vi "DAQ_basics.vi"() -> ()   [LabVIEW 2016]
uses:
  <vilib>/DAQmx/write.llb/DAQmx Write.vi
  <vilib>/DAQmx/write.llb/DAQmx Write (Digital 1D Wfm NChan NSamp).vi
  <vilib>/DAQmx/create/channels.llb/DAQmx Create Channel (DO-Digital Output).vi
  <vilib>/DAQmx/configure/timing.llb/DAQmx Timing (Sample Clock).vi
  <vilib>/DAQmx/create/channels.llb/DAQmx Create Channel (AI-Voltage-Basic).vi
  <vilib>/DAQmx/read.llb/DAQmx Read (Analog Wfm 1Chan NSamp).vi
  <vilib>/Waveform/DWDTOps.llb/DWDT Get Waveform Time Array.vi
panel:
  in  "Pre-sampling (ms)":dbl=300.0 format="%#_13g"
  in  "Stim parameters":T1={"Name"="", "VPs"=[], "Concentrations (ppm)"=[], "Back valve ON delays"=[], "Back valve OFF delays"=[], "Pulse duration (ms)"=250.0, "Step duration (ms)"=2.0, "Sampling rate (Hz)"=20000.0}
  out "data":waveform(dbl)(graph)
  out "error out":errorcluster
  in  "Back valves":tag[](array[tag])
  in  "Odour valves":tag[](array[tag])
  in  "Counter valves":tag[](array[tag])
  in  "error in":errorcluster
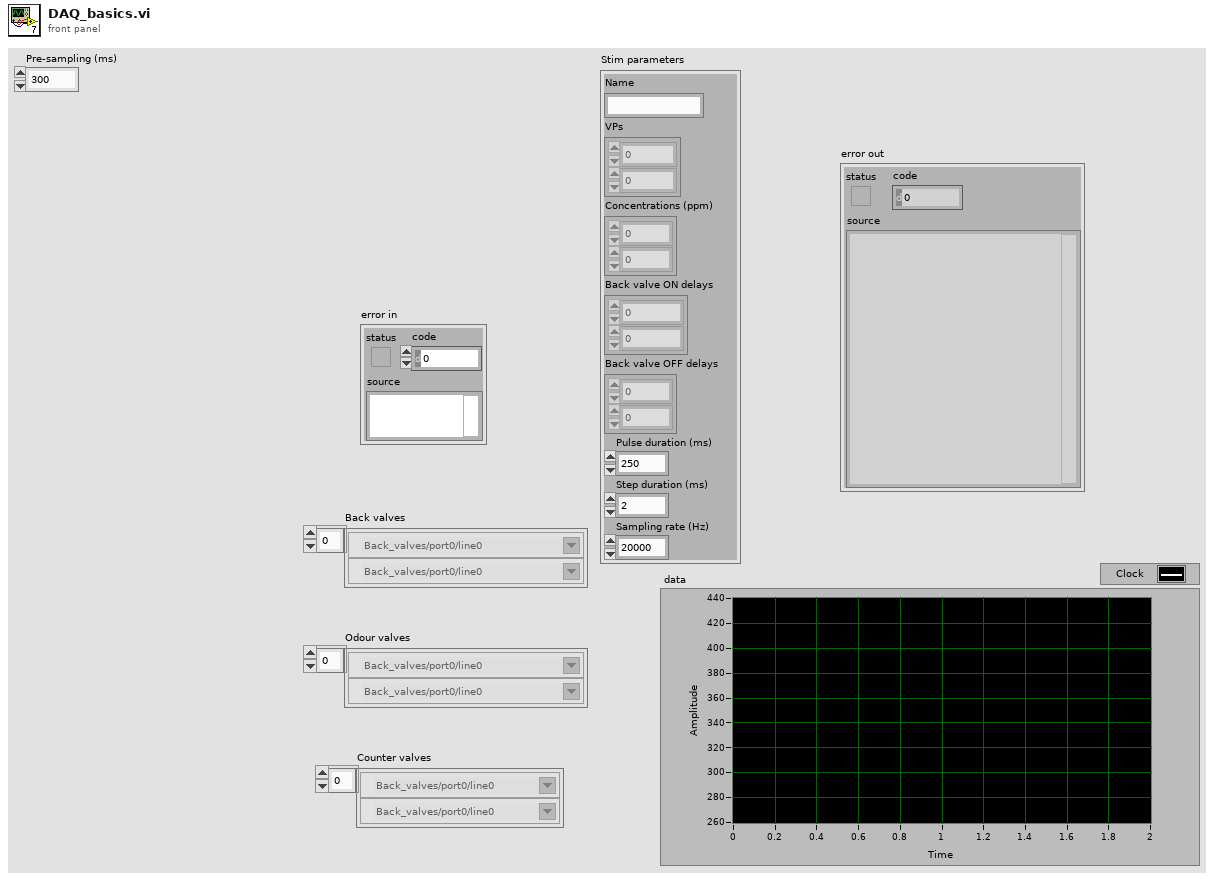
[diagram p1: front panel]
types:
  T1 = cluster{"Name":string, "VPs":dbl[], "Concentrations (ppm)":dbl[], "Back valve ON delays":dbl[], "Back valve OFF delays":dbl[], "Pulse duration (ms)":dbl, "Step duration (ms)":dbl, "Sampling rate (Hz)":dbl}
  T2 = cluster{"VISA Refnum in":refnum<visa-resource-name>, "error in (no error)":errorcluster}
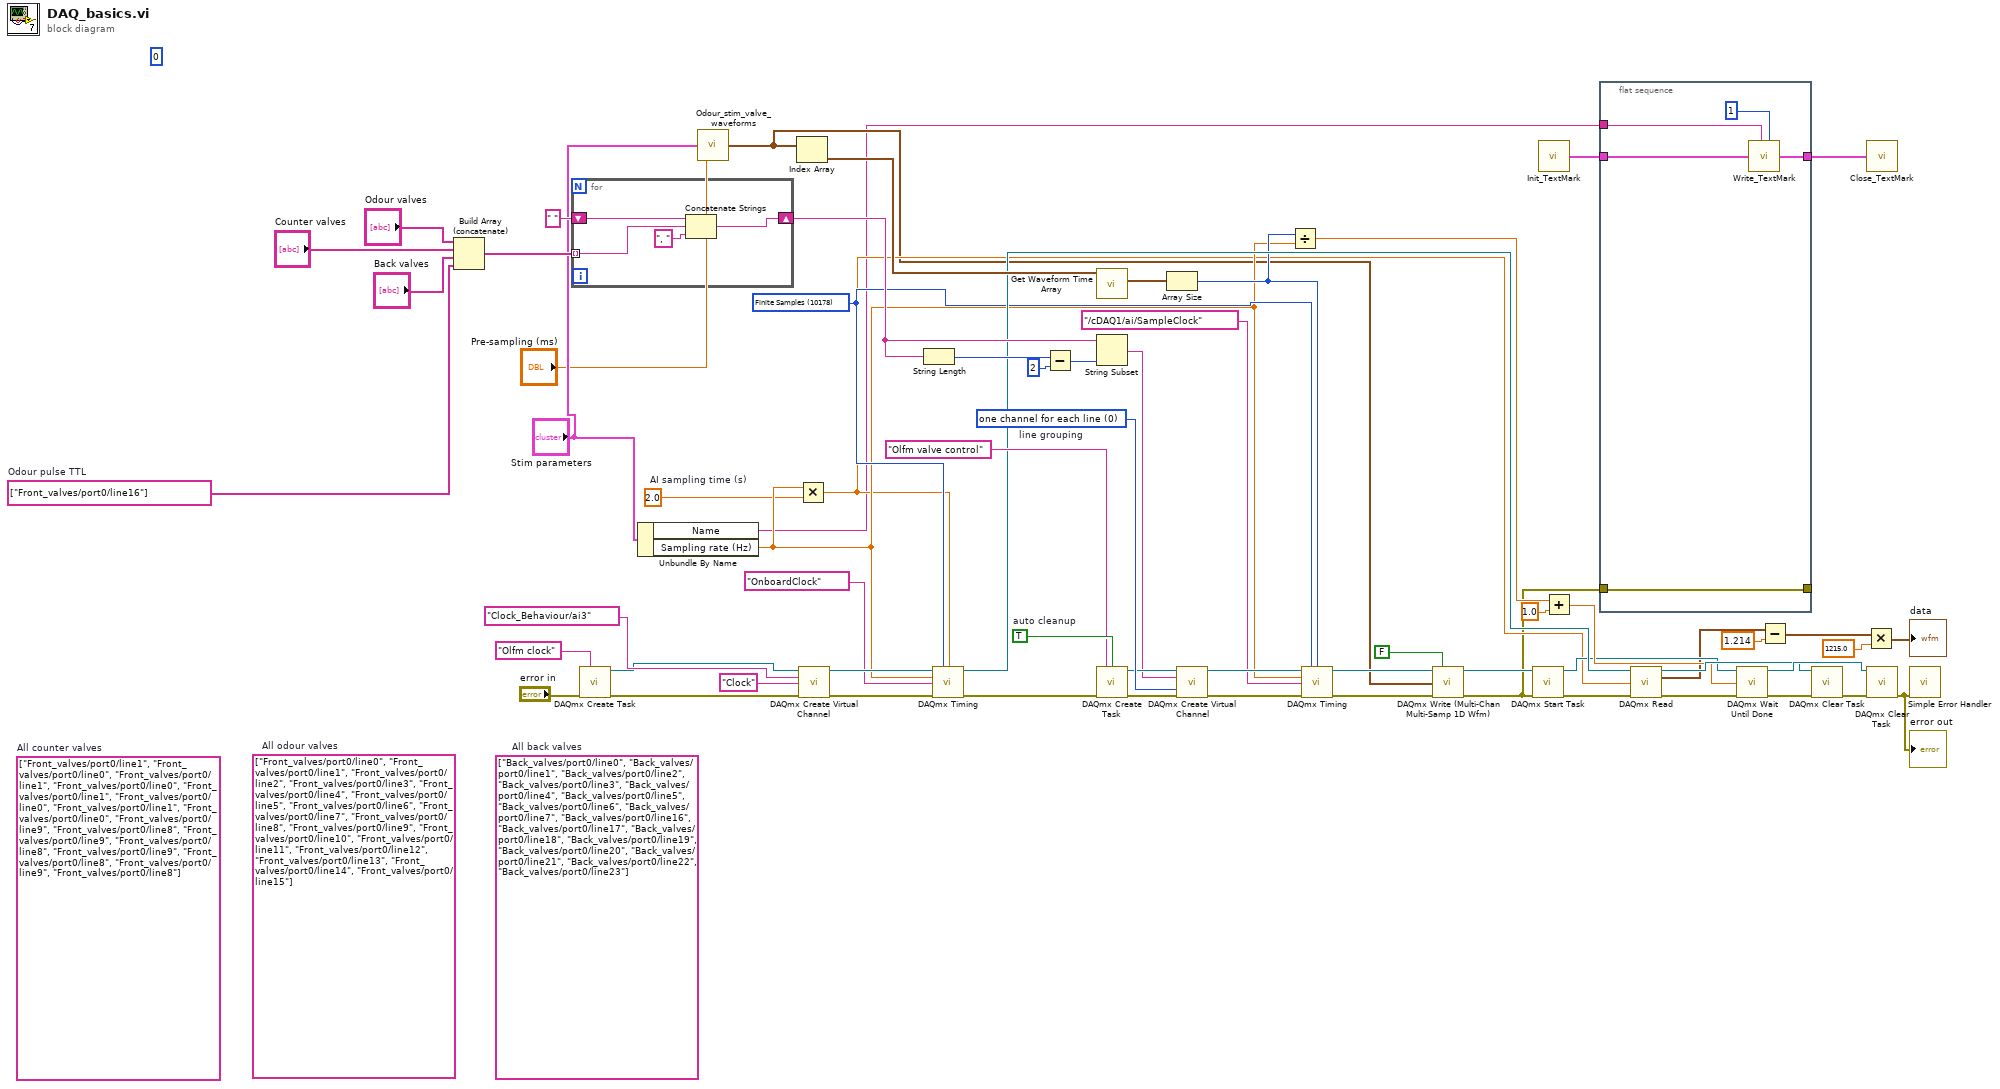
[diagram p0: block diagram]
diagram:
  (unwired) tag[] ["Back_valves/port0/line0", "Back_valves/port0/line1", "Back_valves/port0/line2", "Back_valves/port0/line3", "Back_valves/port0/line4", "Back_valves/port0/line5", "Back_valves/port0/line6", "Back_valves/port0/line7", "Back_valves/port0/line16", "Back_valves/port0/line17", "Back_valves/port0/line18", "Back_valves/port0/line19", "Back_valves/port0/line20", "Back_valves/port0/line21", "Back_valves/port0/line22", "Back_valves/port0/line23"]  # All back valves
  (unwired) tag[] ["Front_valves/port0/line0", "Front_valves/port0/line1", "Front_valves/port0/line2", "Front_valves/port0/line3", "Front_valves/port0/line4", "Front_valves/port0/line5", "Front_valves/port0/line6", "Front_valves/port0/line7", "Front_valves/port0/line8", "Front_valves/port0/line9", "Front_valves/port0/line10", "Front_valves/port0/line11", "Front_valves/port0/line12", "Front_valves/port0/line13", "Front_valves/port0/line14", "Front_valves/port0/line15"]  # All odour valves
  (unwired) tag[] ["Front_valves/port0/line1", "Front_valves/port0/line0", "Front_valves/port0/line1", "Front_valves/port0/line0", "Front_valves/port0/line1", "Front_valves/port0/line0", "Front_valves/port0/line1", "Front_valves/port0/line0", "Front_valves/port0/line9", "Front_valves/port0/line8", "Front_valves/port0/line9", "Front_valves/port0/line8", "Front_valves/port0/line9", "Front_valves/port0/line8", "Front_valves/port0/line9", "Front_valves/port0/line8"]  # All counter valves
  (unwired) 0
  w15 = 2.0  # AI sampling time (s)
  w26 = tag[] ["Front_valves/port0/line16"]  # Odour pulse TTL
  w21 = 10178 items=["Finite Samples"=10178, "Continuous Samples"=10123, "Hardware Timed Single Point"=12522] ("sample mode")
  w62 = 0 items=["one channel for each line", "one channel for all lines"]  # line grouping
  w63 = TRUE  # auto cleanup
  n1 = Build Array (concatenate)("Odour valves", "Counter valves", "Back valves", w26) -> (w59:tag[])
  n2 = for {
    tunnel: w59 -> [w68] mode=indexing
    shift-right: [w65] -> w53
    shift-left: " " ("concatenated string") -> [w66]
    n3 = Concatenate Strings(w66, w68, ", " ("concatenated string")) -> (w65:string)
  }
  n4 = call <vilib>:"DAQmx Create Task.vi"("new task name"="Olfm clock", "error in"="error in") -> ("task out"=w41:refnum<k21>, "error out"=w45:errorcluster)  [unwired: 12 in]
  n5 = Unbundle By Name("Stim parameters") -> ("Name"=w7:string, "Sampling rate (Hz)"=w16:dbl)
  n6 = call "Odour_stim_valve_waveforms.vi"("Odour bottles"="Pre-sampling (ms)", "Olfactormeter parameters"="Stim parameters") -> ("waveform array"=w13:digitalwaveform[])  [unwired: 1 in]
  n7 = Index Array(array=w13) -> (element=w55:digitalwaveform)  [unwired: 1 in]
  n8 = Multiply(x=w16, y=w15) -> (x*y=w14:dbl)
  n9 = call-poly <vilib>:"DAQmx Create Virtual Channel.vi"("task in"=w41, "physical channels"=tag "Clock_Behaviour/ai3", "name to assign"="Clock", "error in"=w45) -> ("task out"=w32:refnum<k21>, "error out"=w31:errorcluster)  [unwired: 10 in]
  n10 = String Length(string=w53) -> (length=w51:i32)
  n11 = call-poly <vilib>:"DAQmx Timing.vi"("task/channels in"=w32, "sample mode"=w21, "samples per channel"=w14, "rate"=w16, "source"=tag "OnboardClock" ("Sample Clock Source"), "error in"=w31) -> ("task out"=w37:refnum<k21>, "error out"=w38:errorcluster)  [unwired: 8 in]
  n12 = Subtract(x=w51, y=2) -> (x-y=w52:i32)
  n13 = call-poly <vilib>:"Get Waveform Time Array.vi"("waveform in"=w55) -> ("X array"=w54:timestamp[])  [unwired: 9 in, 1 out]
  n14 = String Subset(string=w53, length (rest)=w52) -> (substring=w49:string)  [unwired: 1 in]
  n15 = call <vilib>:"DAQmx Create Task.vi"("new task name"="Olfm valve control", "auto cleanup"=w63, "error in"=w38) -> ("task out"=w56:refnum<k21>, "error out"=w39:errorcluster)  [unwired: 11 in]
  n16 = Array Size(array=w54) -> (size(s)=w20:i32)
  n17 = call-poly <vilib>:"DAQmx Create Virtual Channel.vi"("task in"=w56, "lines"=w49, "line grouping"=w62, "error in"=w39) -> ("task out"=w33:refnum<k21>, "error out"=w22:errorcluster)  [unwired: 10 in]
  n18 = Divide(x=w20, y=w16) -> (x/y=w30:dbl)
  n19 = call-poly <vilib>:"DAQmx Timing.vi"("task/channels in"=w33, "sample mode"=w21, "samples per channel"=w20, "rate"=w16, "source"=tag "/cDAQ1/ai/SampleClock", "error in"=w22) -> ("task out"=w23:refnum<k21>, "error out"=w12:errorcluster)  [unwired: 8 in]
  n20 = call-poly "DAQmx Write (Multi-Chan Multi-Samp 1D Wfm).vi"("task/channels in"=w23, "auto start"=FALSE, "data"=w13, "error in"=w12) -> ("task out"=w25:refnum<k21>, "error out"=w6:errorcluster)  [unwired: 9 in, 1 out]
  n21 = call <vilib>:"DAQmx Start Task.vi"("task/channels in"=w25, "error in"=w6) -> ("task out"=w24:refnum<k21>, "error out"=w11:errorcluster)  [unwired: 12 in]
  n22 = call "Init_TextMark.vi"() -> ("TextMark out"=w9:T2)
  n23 = Add(x=w30, y=1.0 ("timeout (s)")) -> (x+y=w28:dbl)
  n24 = flat-sequence {
    tunnel: w6 -> [w73]
    tunnel: [w73] -> _
    tunnel: w9 -> [w72]
    tunnel: [w71] -> w8
    tunnel: w7 -> [w70]
    frame #0 {
      n25 = call "Write_TextMark.vi"("text"=w70, "TextMark in"=w72, "type"=1) -> ("TextMark out"=w71:T2)  [unwired: 6 in]
    }
  }
  n26 = call-poly <vilib>:"DAQmx Read.vi"("task/channels in"=w37, "number of samples per channel"=w14, "error in"=w11) -> ("task out"=w36:refnum<k21>, "data"=w5:waveform(dbl), "error out"=w10:errorcluster)  [unwired: 10 in]
  n27 = call <vilib>:"DAQmx Wait Until Done.vi"("task/channels in"=w24, "timeout (sec)"=w28, "error in"=w10) -> ("task out"=w47:refnum<k21>, "error out"=w35:errorcluster)  [unwired: 11 in]
  n28 = Subtract(x=w5, y=1.214) -> (x-y=w3:waveform(dbl))
  n29 = call <vilib>:"DAQmx Clear Task.vi"("task in"=w36, "error in"=w35) -> ("error out"=w34:errorcluster)  [unwired: 13 in]
  n30 = Multiply(x=w3, y=1215.0) -> (x*y=→"data":waveform(dbl))
  n31 = call "Close_TextMark.vi"("TextMark in"=w8) -> ()
  n32 = call <vilib>:"DAQmx Clear Task.vi"("task in"=w47, "error in"=w34) -> ("error out"=w46:errorcluster)  [unwired: 13 in]
  "error out" <- w46
  n33 = call <vilib>:"Simple Error Handler.vi"("error in (no error)"=w46) -> ()  [unwired: 4 in, 5 out]
